vi "SetDigialFilterState.vi"(8 "Error In":errorcluster, 9 "Enabled?":bool, 10 "Channel (1 or 2)":u8, 11 "Keithley 6482 In":refnum<visa-resource-name>) -> (0 "Error Out":errorcluster, 3 "Keithley 6482 Out":refnum<visa-resource-name>)   [LabVIEW 8.6, in "Keithley-6482-Visa.lvlib"]
uses:
  Keithley-6482-Visa.lvlib
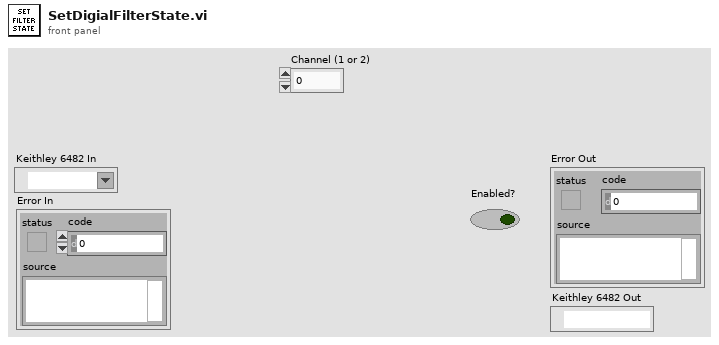
[diagram p1: front panel]
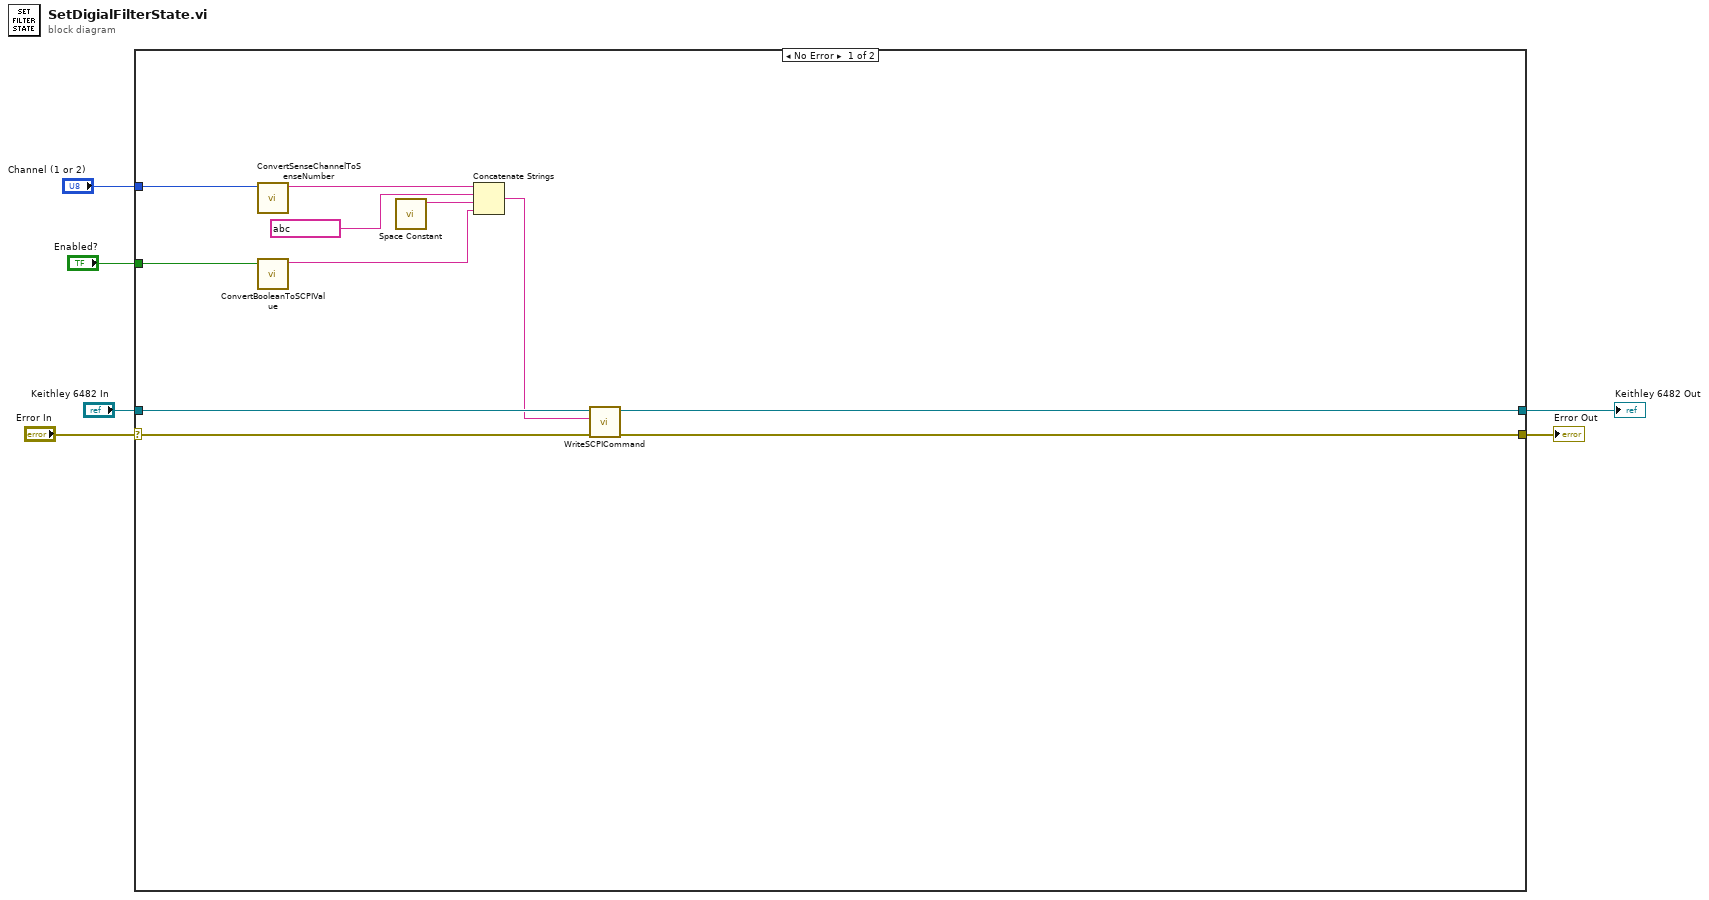
[diagram p0: block diagram]
diagram:
  n1 = case shown="No Error" "Error In" {
    selector: "Error In" -> [w17 w18]
    tunnel: "Keithley 6482 In" -> [w16 w19]
    tunnel: [w9 w18] -> w4
    tunnel: [w10 w19] -> w3
    tunnel: "Channel (1 or 2)" -> [w15 _]
    tunnel: "Enabled?" -> [w7 _]
    frame #0 {
      n2 = call "ConvertSenseChannelToSenseNumber.vi"("Channel (1 or 2)"=w15) -> ("Sense Number"=w14:string)  [unwired: 10 in]
      n3 = call "ConvertBooleanToSCPIValue.vi"("Boolean"=w7) -> ("SCPI Value"=w8:string)  [unwired: 10 in]
      n4 = call <vilib>:"Space Constant.vi"() -> ("String"=w12:string)
      n5 = Concatenate Strings(w14, string ? ("string"), w12, w8) -> (w11:string)
      n6 = call "WriteSCPICommand.vi"("Error In"=w17, "SCPI Command"=w11, "Keithley 6482 In"=w16) -> ("Error Out"=w9:errorcluster, "Keithley 6482 Out"=w10:refnum<visa-resource-name>)  [unwired: 7 in]
    }
    frame #1 {
    }
  }
  "Error Out" <- w4
  "Keithley 6482 Out" <- w3
